vi "Read Transfer Group Buffer.vi"(8 "error in":errorcluster, 10 "Transfer Group":refnum<class "Transfer Group.lvclass">, 11 "RDMA Transceiver in":refnum<class "RDMA Transceiver.lvclass">) -> (0 "error out":errorcluster, 1 "data":string, 3 "RDMA Transceiver out":refnum<class "RDMA Transceiver.lvclass">)   [LabVIEW 2020, in "RDMA.lvlib" / "RDMA Transceiver.lvclass"]
uses:
  RDMA Transceiver.lvclass
  DSF Core.lvlibp/Classes/Transfer Group/Transfer Group.lvclass
  DSF Core.lvlibp/Classes/Buffer/Buffer.lvclass
  DSF Core.lvlibp/Classes/Buffer/Read Buffer 1D U8.vi
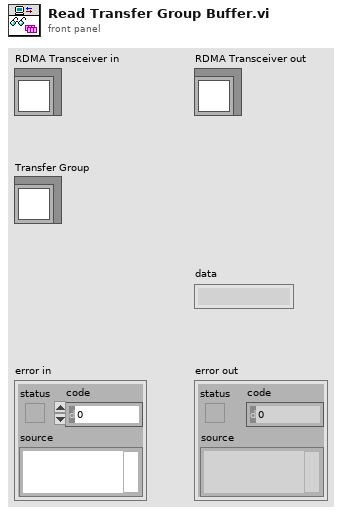
[diagram p1: front panel]
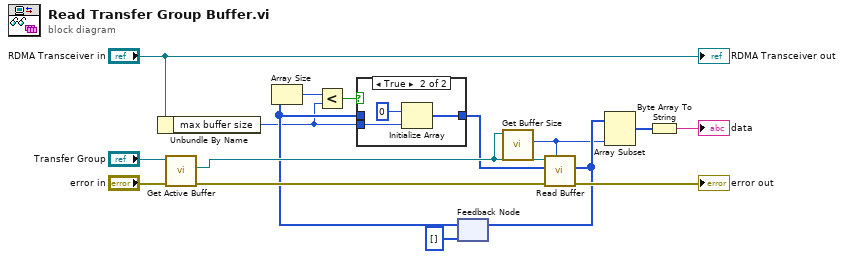
[diagram p0: block diagram]
diagram:
  n1 = Unbundle By Name("RDMA Transceiver in") -> ("max buffer size"=w1:i32)
  n2 = call "Get Active Buffer.vi"("error in (no error)"="error in", "Transfer Group in"="Transfer Group") -> ("error out"=w12:errorcluster, "Buffer"=w8:refnum<class "Buffer.lvclass">)  [unwired: 7 in, 1 out]
  n3 = feedback #1(u8[] []) -> (w2:u8[])
  n4 = Array Size(array=w2) -> (size(s)=w4:i32)
  n5 = Less?(x=w4, y=w1) -> (x < y?=w3:bool)
  n6 = case shown="True" w3 {
    tunnel: w2 -> [w17 _]
    tunnel: [w17 w20] -> w7
    tunnel: w1 -> [_ w18]
    frame False {
    }
    frame True {
      n7 = Initialize Array(u8 0 ("Numeric"), w18) -> (w20:u8[])
    }
  }
  n8 = call "Get Buffer Size.vi"("Buffer in"=w8) -> ("buffer size"=w5:u64)  [unwired: 9 in, 1 out]
  n9 = call-poly "Read Buffer.vi"("count (-1: rest)"=w5, "error in (no error)"=w12, "dst array in"=w7, "Buffer in"=w8) -> ("error out"=→"error out":errorcluster, "dst array out"=w6:u8[])  [unwired: 4 in, 2 out]
  n10 = feedback-in #1(w6) -> ()
  n11 = Array Subset(array=w6, length=w5) -> (w14:u8[])  [unwired: 1 in]
  n12 = Byte Array To String(unsigned byte array=w14) -> (string=→"data":string)
  "RDMA Transceiver out" <- "RDMA Transceiver in"
